vi "Pointer.Offset by Type.vi"(7 "data type":T1, 10 "count (1)":i64=1, 11 "pointer":u64 format="%016x") -> (3 "offset pointer":u64 format="%016x")   [LabVIEW 2016, in "VeriStand Data.lvlib"]
doc: "Offsets the provided <B>pointer</B> by the size, in bytes, determined by <B>count</B> and <B>data type</B>."
uses:
  VeriStand Data.lvlib
  Typedefs/Typedefs.Data Types.ctl
  Utilities/Utilities.Sizeof.Scalar.vi
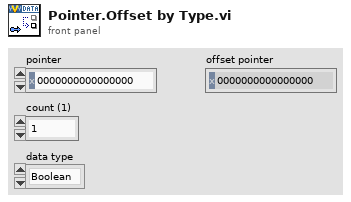
[diagram p1: front panel]
types:
  T1 = typedef "VeriStand Data.lvlib/Typedefs.Data Types.ctl" = enum16{"Boolean", "Single", "Double", "I8", "I16", "I32", "I64", "U8", "U16", "U32", "U64"}
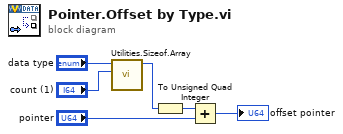
[diagram p0: block diagram]
diagram:
  n1 = call "Utilities.Sizeof.Array.vi"("count"="count (1)", "data type"="data type") -> ("size"=w2:u64)  [unwired: 9 in]
  n2 = To Unsigned Quad Integer(1:w2) -> (0:w1:u64)
  n3 = Add(x=w1, y="pointer") -> (x+y=→"offset pointer":u64)
